vi "RSZVB Configure Trigger Periodic.vi"(8 "error in (no error)":errorcluster {"code" format="%.0x"}, 9 "Trigger Period (1.0 s)":dbl=1.0 format="%^.3e", 10 "Channel (1)":i32=1, 11 "VISA session":refnum<visa-resource-name>) -> (0 "error out":errorcluster {"code" format="%.0x"}, 3 "dup VISA session":refnum<visa-resource-name>)   [LabVIEW 2011]
doc: "This VI configures the periodic trigger mode. In Periodic trigger mode the measurement is triggered by the periodic signal of an internal clock generator.\n\nRemote-control command(s):\nTRIGger<Ch>[:SEQuence]:SOURce TIMer\nTRIGger<Ch>[:SEQuence]:TIMer"
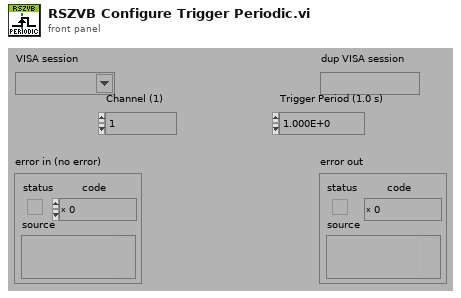
[diagram p1: front panel]
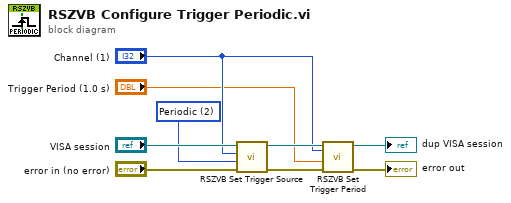
[diagram p0: block diagram]
diagram:
  w1 = 2 items=["Free Run", "External", "Periodic", "Manual", "RF Power"] ("Trigger Source (0: Free Run)")
  n1 = call "RSZVB Set Trigger Source.vi"("error in (no error)"="error in (no error)", "Trigger Source (0: Free Run)"=w1, "Channel (1)"="Channel (1)", "VISA session"="VISA session") -> ("error out"=w7:errorcluster, "dup VISA session"=w6:refnum<visa-resource-name>)  [unwired: 6 in]
  n2 = call "RSZVB Set Trigger Period.vi"("error in (no error)"=w7, "Trigger Period (1.0 s)"="Trigger Period (1.0 s)", "Channel (1)"="Channel (1)", "VISA session"=w6) -> ("error out"=→"error out":errorcluster, "dup VISA session"=→"dup VISA session":refnum<visa-resource-name>)  [unwired: 6 in]
